vi "init multiclamp_N.vi"(5 "channels to initialize":T2(array[ring])=[enum."manipulator 1", enum."manipulator 2"], 8 "error in (no error)":errorcluster, 11 "holding V (mV)":dbl=-70.0) -> (0 "error out":errorcluster, 1 "Error out":i32, 2 "mclamp cluster out":T1, 3 "Multiclamp Handle Out":u32=722860)   [LabVIEW 2015]
uses:
  multiBot/patcherBot/AxMultiClampMsg.dll
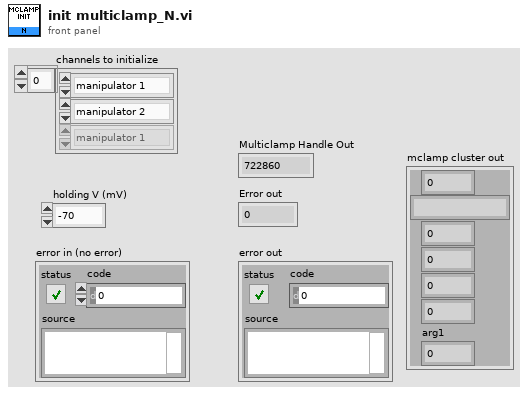
[diagram p1: front panel]
types:
  T1 = cluster{u32, string, i32, u32, u32, u32, "arg1":i32}
  T2 = enum16{"manipulator 1", "manipulator 2", "manipulator 3", "manipulator 4"}[]
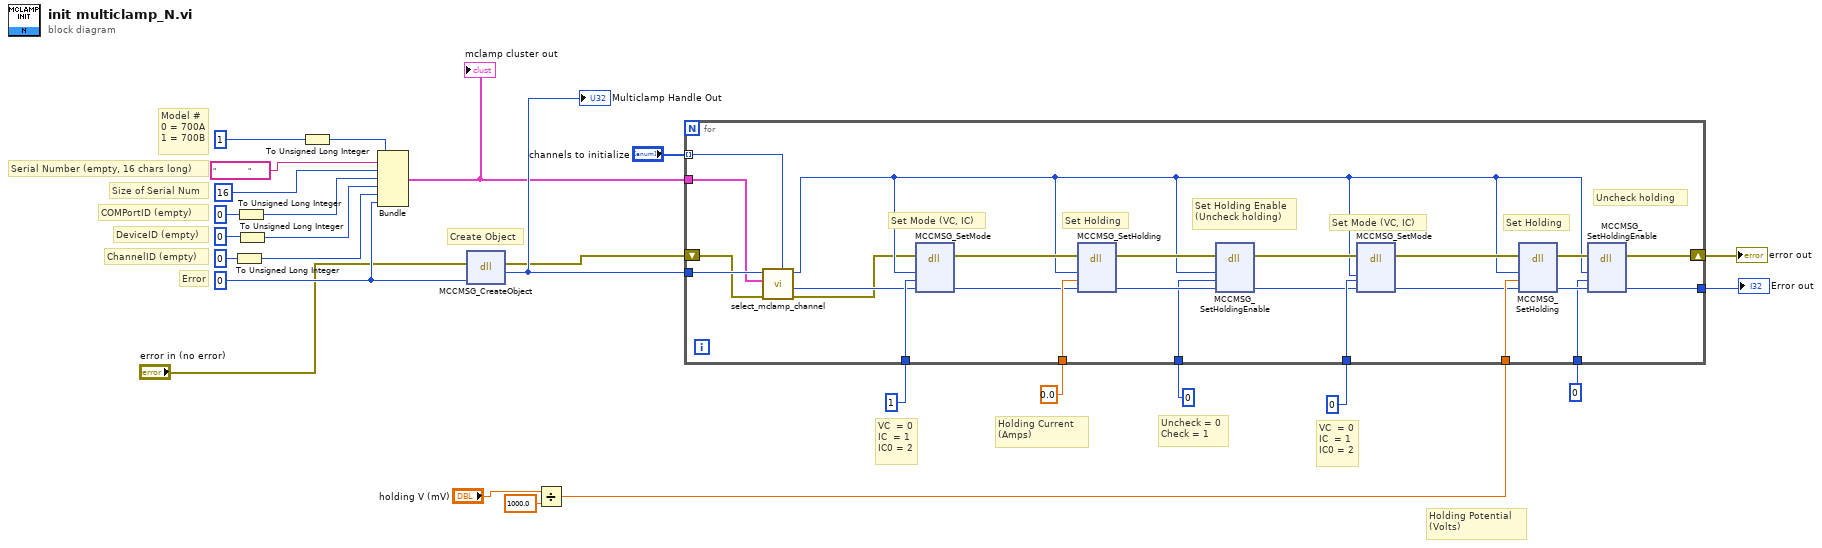
[diagram p0: block diagram]
diagram:
  w17 = 0 ("arg1")
  # "Holding Current \n(Amps)"
  # "Uncheck = 0\nCheck = 1"
  # "VC  = 0\nIC  = 1\nIC0 = 2"
  # "Holding Potential \n(Volts)"
  # "VC  = 0\nIC  = 1\nIC0 = 2"
  # "Error"
  # "ChannelID (empty)"
  # "DeviceID (empty)"
  # "COMPortID (empty)"
  # "Size of Serial Num"
  # "Serial Number (empty, 16 chars long)"
  # "Model #\n0 = 700A\n1 = 700B"
  # "Create Object"
  n1 = To Unsigned Long Integer(number=u32 0) -> (unsigned 32bit integer=w23:u32)
  n2 = To Unsigned Long Integer(number=u32 0) -> (unsigned 32bit integer=w25:u32)
  n3 = To Unsigned Long Integer(number=u32 0) -> (unsigned 32bit integer=w24:u32)
  n4 = To Unsigned Long Integer(number=u32 1) -> (unsigned 32bit integer=w26:u32)
  n5 = Bundle(w26, "                ", 16, w25, w24, w23, "arg1"=w17) -> (w5:T1)  [unwired: 1 in]
  "mclamp cluster out" <- w5
  n6 = dll-call lib="C:/multiBot/patcherBot/AxMultiClampMsg.dll" fn="MCCMSG_CreateObject"(error in="error in (no error)", "error"=w17) -> (error out=w6:errorcluster, "return type"=w7:u32)  [unwired: 3 in, 1 out]
  "Multiclamp Handle Out" <- w7
  n7 = Divide(x="holding V (mV)", y=1000.0) -> (x/y=w10:dbl)
  n8 = for {
    tunnel: u32 0 ("number") -> [w51]
    tunnel: 0.0 ("ModeConstant") -> [w50]
    tunnel: u32 1 ("number") -> [w49]
    tunnel: w10 -> [w43]
    tunnel: w7 -> [w41]
    tunnel: w5 -> [w31]
    shift-right: [w42] -> w8
    shift-left: w6 -> [w37]
    tunnel: 0 ("ModeConstant") -> [w30]
    tunnel: 0 ("ModeConstant") -> [w29]
    tunnel: "channels to initialize" -> [w28] mode=indexing
    tunnel: [w27] -> w1
    # "Uncheck holding"
    # "Set Holding Enable\n(Uncheck holding)"
    # "Set Holding"
    # "Set Mode (VC, IC)"
    # "Set Holding"
    # "Set Mode (VC, IC)"
    n9 = call "select_mclamp_channel.vi"("which manipulator"=w28, "error in (no error)"=w37, "mclamp cluster"=w31, "Multiclamp Handle In"=w41) -> ("error out"=w38:errorcluster, "error"=w39:i32, "Multiclamp Handle out"=w40:u32)  [unwired: 5 in]
    n10 = dll-call lib="C:/multiBot/patcherBot/AxMultiClampMsg.dll" fn="MCCMSG_SetMode"(error in=w38, "handle"=w40, "ModeConstant"=w49, "error"=w39) -> (error out=w48:errorcluster, "error"=w36:i32)  [unwired: 5 in, 1 out]
    n11 = dll-call lib="C:/multiBot/patcherBot/AxMultiClampMsg.dll" fn="MCCMSG_SetHolding"(error in=w48, "handle"=w40, "ModeConstant"=w50, "error"=w36) -> (error out=w47:errorcluster, "error"=w32:i32)  [unwired: 5 in, 1 out]
    n12 = dll-call lib="C:/multiBot/patcherBot/AxMultiClampMsg.dll" fn="MCCMSG_SetHoldingEnable"(error in=w47, "handle"=w40, "ModeConstant"=w29, "error"=w32) -> (error out=w46:errorcluster, "error"=w33:i32)  [unwired: 5 in, 1 out]
    n13 = dll-call lib="C:/multiBot/patcherBot/AxMultiClampMsg.dll" fn="MCCMSG_SetMode"(error in=w46, "handle"=w40, "ModeConstant"=w51, "error"=w33) -> (error out=w45:errorcluster, "error"=w34:i32)  [unwired: 5 in, 1 out]
    n14 = dll-call lib="C:/multiBot/patcherBot/AxMultiClampMsg.dll" fn="MCCMSG_SetHolding"(error in=w45, "handle"=w40, "ModeConstant"=w43, "error"=w34) -> (error out=w44:errorcluster, "error"=w35:i32)  [unwired: 5 in, 1 out]
    n15 = dll-call lib="C:/multiBot/patcherBot/AxMultiClampMsg.dll" fn="MCCMSG_SetHoldingEnable"(error in=w44, "handle"=w40, "ModeConstant"=w30, "error"=w35) -> (error out=w42:errorcluster, "error"=w27:i32)  [unwired: 5 in, 1 out]
  }
  "Error out" <- w1
  "error out" <- w8
